vi "Calc Value.vi"(8 "error in (no error)":errorcluster, 11 "PV Calc in":refnum<class "PV Calc.lvclass">) -> (0 "error out":errorcluster, 2 "Value":dbl, 3 "PV Calc out":refnum<class "PV Calc.lvclass">)   [LabVIEW 2020, in "VolatusControl.lvlib" / "PV Calc.lvclass"]
uses:
  PV Calc.lvclass
  PV Calc.lvclass/PV Calc.ctl
  lv-vecto/Vecto/Channel DBL/Channel DBL.lvclass
  <vilib>/Analysis/NI_AALBase.lvlib
  <vilib>/Analysis/baseanly.llb/Mean (DBL).vi
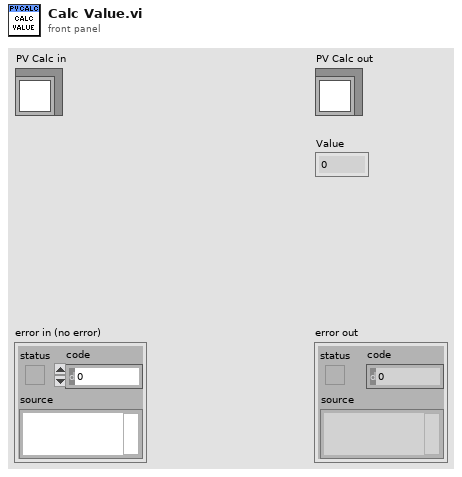
[diagram p1: front panel]
types:
  T1 = typedef "VolatusControl.lvlib/PV Calc.lvclass/Calc Type.ctl" = enum16{"Average", "Median", "Min", "Max"}
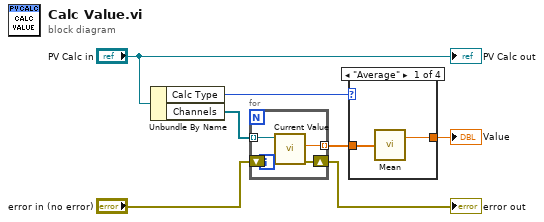
[diagram p0: block diagram]
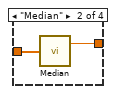
[diagram p2: hidden frame]
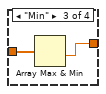
[diagram p3: hidden frame]
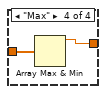
[diagram p4: hidden frame]
diagram:
  n1 = Unbundle By Name("PV Calc in") -> ("Calc Type"=w5:T1, "Channels"=w6:refnum<class "Channel DBL.lvclass">[])
  n2 = for {
    tunnel: w6 -> [w11] mode=indexing
    tunnel: [w10] -> w4 mode=indexing
    shift-right: [w9] -> w1
    shift-left: "error in (no error)" -> [w8]
    n3 = call "Current Value.vi"("error in (no error)"=w8, "Channel in"=w11) -> ("error out"=w9:errorcluster, "Scaled"=w10:dbl)  [unwired: 5 in, 3 out]
  }
  "error out" <- w1
  n4 = case shown="\"Average\"" w5 {
    tunnel: w4 -> [w13 w15 w17 w19]
    tunnel: [w12 w14 w16 w18] -> w3
    frame "Average" {
      n5 = call-poly <vilib>:"Mean.vi"("X"=w13) -> ("mean"=w12:dbl)  [unwired: 1 out]
    }
    frame "Median" {
      n6 = call <vilib>:"Median.vi"("X"=w15) -> ("median"=w14:dbl)  [unwired: 1 out]
    }
    frame "Min" {
      n7 = Array Max & Min(array=w17) -> (min value=w16:dbl)  [unwired: 3 out]
    }
    frame "Max" {
      n8 = Array Max & Min(array=w19) -> (max value=w18:dbl)  [unwired: 3 out]
    }
  }
  "Value" <- w3
  "PV Calc out" <- "PV Calc in"
